vi "GetCXT.vi"(5 "format string (%_20f)":string="%_20f", 7 "key description":string, 8 "sections":string[](array[string]), 9 "numeric":cxt, 11 "info data":string) -> (0 "sections out":string[](array[string]), 2 "value":cxt format="%#_20g", 3 "info data out":string)   [LabVIEW 2019, in "infolib.lvlib"]
doc: "Add a new numeric key to Info Data string. If section exists in Info Data string, inserts key into this section."
uses:
  infolib.lvlib
panel:
  out "value 3":ext
  out "value 2":ext
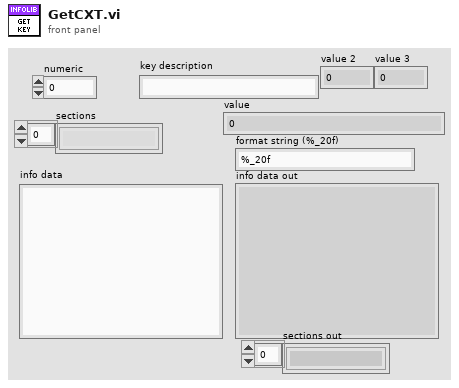
[diagram p1: front panel]
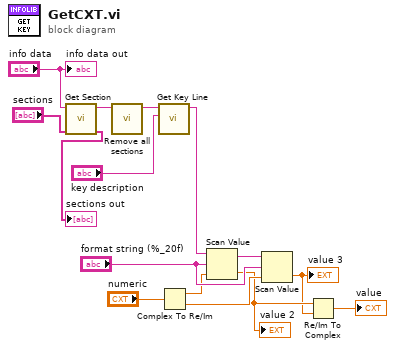
[diagram p0: block diagram]
diagram:
  n1 = call "Get Section.vi"("sections"="sections", "info data"="info data") -> ("sections out"=→"sections out":string[], "section part"=w15:string)  [unwired: 7 in, 1 out]
  n2 = call "Remove all sections.vi"("info data"=w15) -> ("info data out"=w14:string)  [unwired: 10 in]
  n3 = call "Get Key Line.vi"("key description"="key description", "info data"=w14) -> ("key value"=w11:string)  [unwired: 9 in]
  n4 = Complex To Re/Im(x + iy="numeric") -> (x=w7:ext, y=w6:ext)
  n5 = Scan Value(string=w11, format string="format string (%_20f)", default (0 dbl)=w7) -> (output string=w10:string, value=w5:ext)
  "value 2" <- w5
  n6 = Scan Value(string=w10, format string="format string (%_20f)", default (0 dbl)=w6) -> (value=w4:ext)  [unwired: 1 out]
  "value 3" <- w4
  n7 = Re/Im To Complex(1:w4, 2:w5) -> (0:→"value":cxt)
  "info data out" <- "info data"
